vi "Get_Data_Base_file_code.vi"(0 "Results Filename":path, 1 "Data Type":string="Measurement") -> (2 "DB file code":string, 3 "Raw Data Folder":string, 4 "Raw Data File Name":path, 5 "Raw Data File Number":string)   [LabVIEW 2010]
uses:
  Get_File_Code_case.ctl
  Controls/Post_Process.ctl
  Globals/Constants_global.vi
  Globals/Trav_pos_global.vi
  Globals/Meas_global.vi
panel:
  out "File Code Case":T1
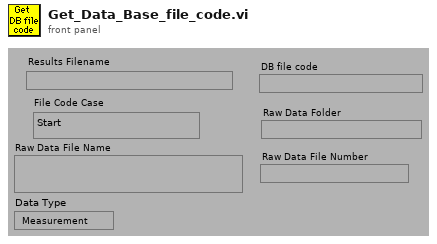
[diagram p1: front panel]
types:
  T1 = typedef "Get_File_Code_case.ctl" = enum16{"Start", "Read DB info file", "Does Results file already exist", "Create DB info directory", "Add file to list", "Write DB info file", "End"}
  T2 = typedef "Post_Process.ctl" = enum16{"Take New Data", "Post Process Raw Data File"}
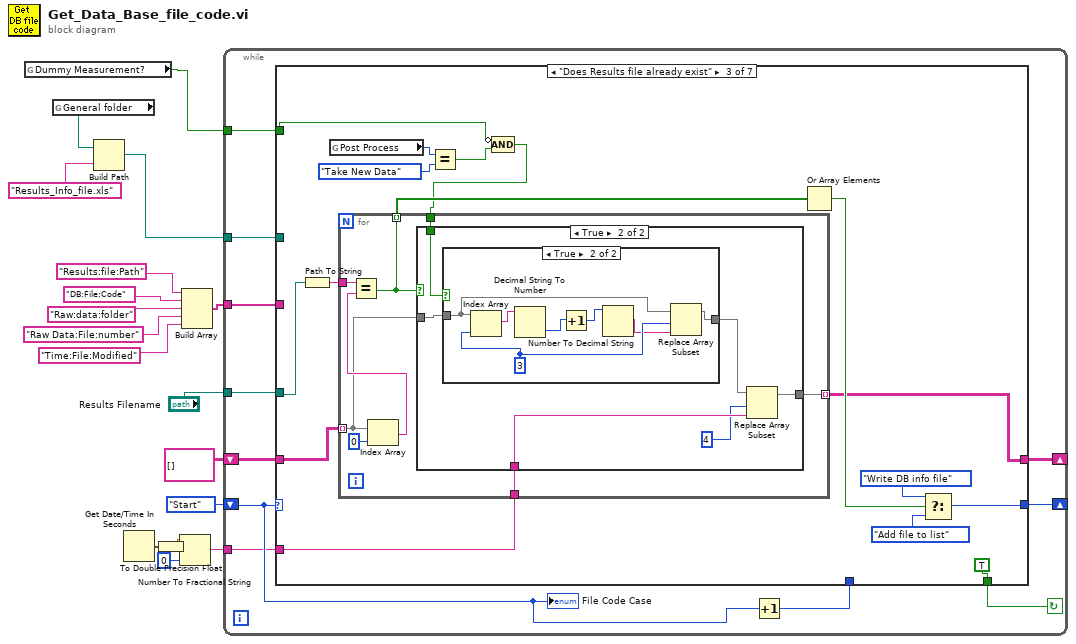
[diagram p0: block diagram]
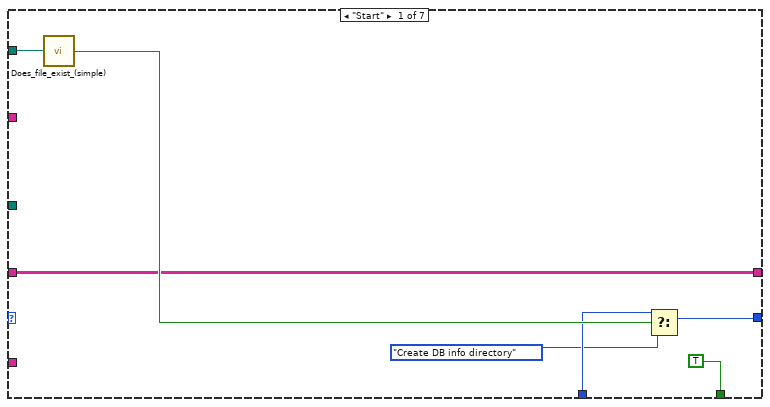
[diagram p2: hidden frame]
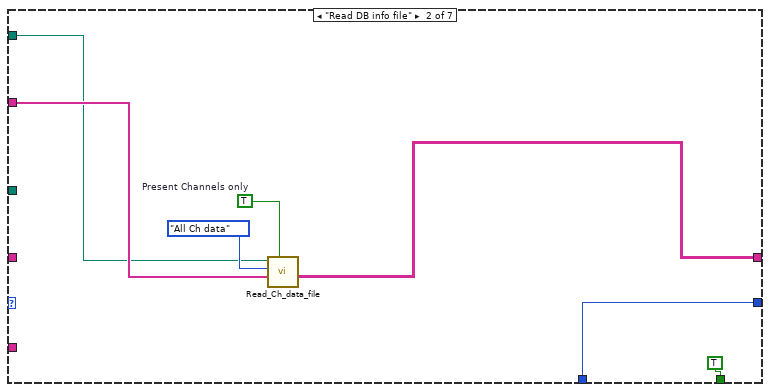
[diagram p3: hidden frame]
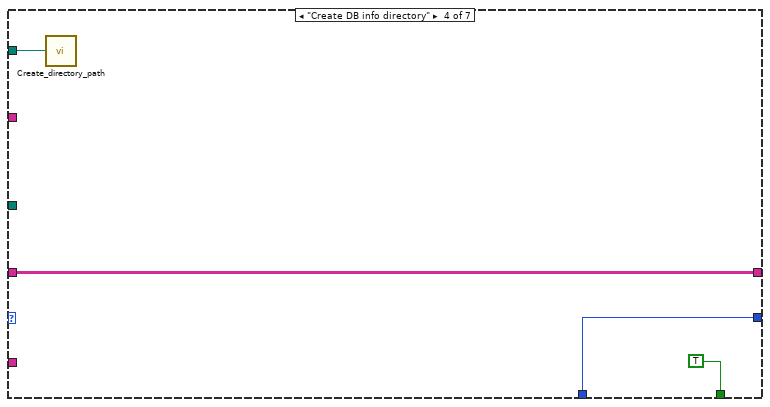
[diagram p6: hidden frame]
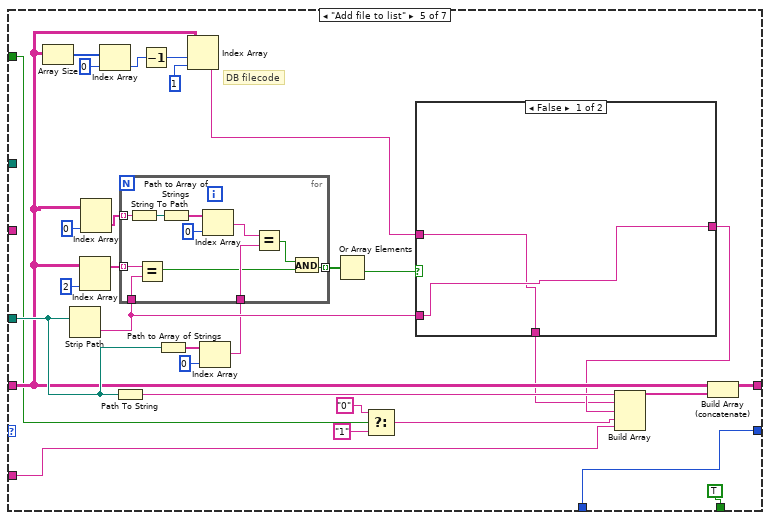
[diagram p7: hidden frame]
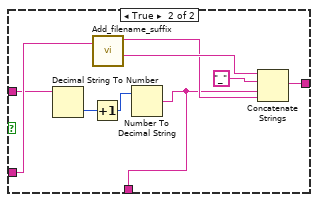
[diagram p8: hidden frame]
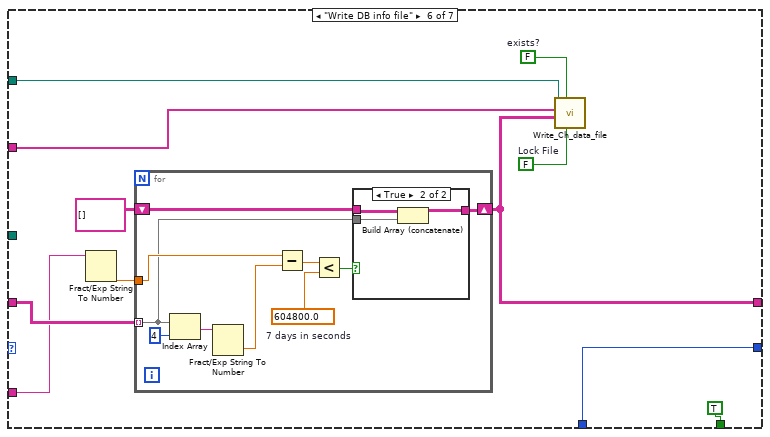
[diagram p9: hidden frame]
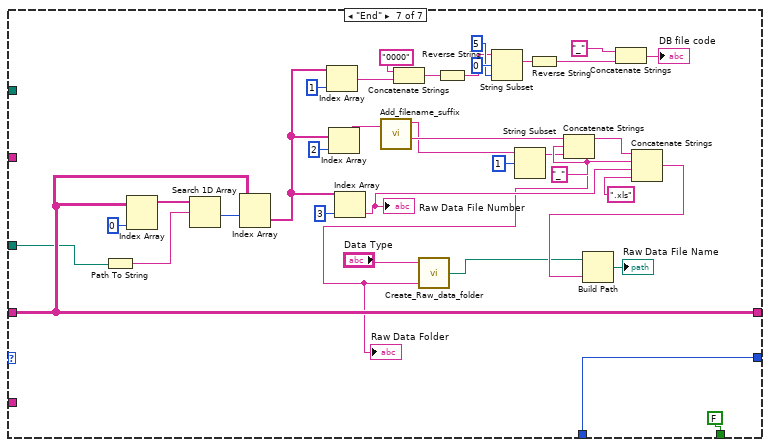
[diagram p11: hidden frame]
diagram:
  n1 = global read "Trav_pos_global.vi" "Dummy Measurement?"() -> (w1:bool)
  n2 = global read "Constants_global.vi" "General folder"() -> (w7:path)
  n3 = Build Path(base path=w7, name or relative path="Results_Info_file.xls" ("Substring")) -> (appended path=w6:path)
  n4 = Get Date/Time In Seconds() -> (seconds since 1Jan1904=w2:timestamp)
  n5 = To Double Precision Float(number=w2) -> (double precision float=w4:dbl)
  n6 = Number To Fractional String(number=w4, precision (6)=i16 0) -> (F-format string=w3:string)  [unwired: 2 out]
  n7 = Build Array("Results:file:Path", "DB:File:Code", "Raw:data:folder", "Raw Data:File:number", "Time:File:Modified") -> (w11:string[])
  n8 = while {
    tunnel: w3 -> [w19]
    tunnel: w11 -> [w20]
    tunnel: "Results Filename" -> [w22]
    shift-left: string[][] [] ("2D data array") -> [w21]
    shift-right: [w23] -> _
    tunnel: w6 -> [w24]
    shift-left: Get_File_Code_case."Start" ("File Code Case") -> [w27]
    shift-right: [w25] -> _
    tunnel: w1 -> [w18]
    stop <- w28 continue-if-true
    n9 = Increment(x=w27) -> (x+1=w26:T1)
    n10 = case shown="\"Does Results file already exist\"" w27 {
      tunnel: [TRUE TRUE TRUE TRUE TRUE TRUE FALSE] -> w28
      tunnel: w26 -> [w32 w42 _ w84 w107 w148 w197]
      tunnel: [w30 w42 w52 w84 w107 w148 w197] -> w25
      tunnel: w24 -> [w34 w36 _ w83 _ w145 _]
      tunnel: [w29 w37 w51 w82 w108 w139 w192] -> w23
      tunnel: w22 -> [_ _ w57 _ w101 _ w179]
      tunnel: w21 -> [w29 _ w58 w82 w96 w143 w192]
      tunnel: w20 -> [_ w40 _ _ _ w146 _]
      tunnel: w19 -> [_ _ w49 _ w105 w142 _]
      tunnel: w18 -> [_ _ w43 _ w92 _ _]
      frame "Start" {
        n11 = call "Does_file_exist_(simple).vi"("Pathname"=w34) -> ("exists?"=w33:bool)
        n12 = Select(t=w32, s=w33, f=Get_File_Code_case."Create DB info directory" ("File Code Case")) -> (s? t:f=w30:T1)
      }
      frame "Read DB info file" {
        w38 = TRUE  # Present Channels only
        n13 = call "Read_Ch_data_file.vi"("Present Channels only"=w38, "Present Channels"=w40, "Output"=enum16{"All Ch data", "The last few rows"}."All Ch data", "Filename"=w36) -> ("Channel Values"=w37:string[][])  [unwired: 1 in, 4 out]
      }
      frame "Does Results file already exist" {
        n14 = Path To String(path=w57) -> (string=w48:string)
        n15 = global read "Meas_global.vi" "Post Process"() -> (w46:T2)
        n16 = Equal?(x=w46, y=Post_Process."Take New Data" ("Post Process")) -> (x = y?=w45:bool)
        n17 = Compound Arithmetic op=AND(invert w43, w45) -> (w44:bool)
        n18 = for {
          tunnel: w58 -> [w63] mode=indexing
          tunnel: w48 -> [w65]
          tunnel: [w62] -> w56 mode=indexing
          tunnel: [w61] -> w51 mode=indexing
          tunnel: w49 -> [w60]
          tunnel: w44 -> [w59]
          n19 = Index Array(array=w63, index=0 ("Index")) -> (element=w64:string)
          n20 = Equal?(x=w65, y=w64) -> (x = y?=w62:bool)
          n21 = case shown="True" w62 {
            tunnel: w63 -> [w67 w73]
            tunnel: [w67 w69] -> w61
            tunnel: w60 -> [_ w71]
            tunnel: w59 -> [_ w68]
            frame False {
            }
            frame True {
              n22 = case shown="True" w68 {
                tunnel: w73 -> [w74 w75]
                tunnel: [w74 w77] -> w72
                frame False {
                }
                frame True {
                  w81 = 3 ("Index")
                  n23 = Index Array(array=w75, index=w81) -> (element=w80:string)
                  n24 = Decimal String To Number(string=w80) -> (number=w79:i32)  [unwired: 3 out]
                  n25 = Increment(x=w79) -> (x+1=w78:i32)
                  n26 = Number To Decimal String(number=w78) -> (decimal integer string=w76:string)  [unwired: 1 out]
                  n27 = Replace Array Subset(array=w75, new element=w76, index=w81) -> (w77:string[])
                }
              }
              n28 = Replace Array Subset(array=w72, new element=w71, index=4 ("Index")) -> (w69:string[])
            }
          }
        }
        n29 = Or Array Elements(Boolean array=w56) -> (logical OR=w55:bool)
        n30 = Select(t=Get_File_Code_case."Write DB info file" ("File Code Case"), s=w55, f=Get_File_Code_case."Add file to list" ("File Code Case")) -> (s? t:f=w52:T1)
      }
      frame "Create DB info directory" {
        n31 = call "Create_directory_path.vi"("Path name"=w83) -> ()  [unwired: 1 out]
      }
      frame "Add file to list" {
        # "DB filecode"
        n32 = Array Size(array=w96) -> (size(s)=w113:i32[])
        n33 = Strip Path(path=w101) -> (name=w99:string)  [unwired: 1 out]
        n34 = Index Array(array=w96, index (col)=2) -> (element=w98:string[])  [unwired: 1 in]
        n35 = Index Array(array=w96, index (col)=0) -> (element=w97:string[])  [unwired: 1 in]
        n36 = Index Array(array=w113, index=0) -> (element=w112:i32)
        n37 = Path To String(path=w101) -> (string=w104:string)
        n38 = Decrement(x=w112) -> (x-1=w111:i32)
        n39 = Path to Array of Strings(0:w101) -> (2:w102:string[])  [unwired: 1 out]
        n40 = Index Array(array=w96, index (row)=w111, index (col)=1) -> (element=w87:string)
        n41 = Index Array(array=w102, index=0 ("Index")) -> (element=w95:string)
        n42 = for {
          tunnel: w99 -> [w126]
          tunnel: w98 -> [w125] mode=indexing
          tunnel: w97 -> [w121] mode=indexing
          tunnel: w95 -> [w119]
          tunnel: [w116] -> w94 mode=indexing
          n43 = String To Path(string=w121) -> (path=w122:path)
          n44 = Equal?(x=w125, y=w126) -> (x = y?=w117:bool)
          n45 = Path to Array of Strings(0:w122) -> (2:w123:string[])  [unwired: 1 out]
          n46 = Index Array(array=w123, index=0 ("Index")) -> (element=w120:string)
          n47 = Equal?(x=w120, y=w119) -> (x = y?=w118:bool)
          n48 = And(x=w118, y=w117) -> (x .and. y?=w116:bool)
        }
        n49 = Or Array Elements(Boolean array=w94) -> (logical OR=w93:bool)
        n50 = Select(t="0", s=w92, f="1") -> (s? t:f=w89:string)
        n51 = case shown="False" w93 {
          tunnel: w87 -> [w127 w130]
          tunnel: [w128 w137] -> w88
          tunnel: w99 -> [w128 w135]
          tunnel: [w127 w129] -> w86
          frame False {
          }
          frame True {
            n52 = Decimal String To Number(string=w130) -> (number=w131:i32)  [unwired: 3 out]
            n53 = Increment(x=w131) -> (x+1=w132:i32)
            n54 = call "Add_filename_suffix.vi"("Filename"=w135) -> ("Original Suffix"=w133:string, "Base name"=w134:string)  [unwired: 1 in, 2 out]
            n55 = Number To Decimal String(number=w132) -> (decimal integer string=w129:string)  [unwired: 1 out]
            n56 = Concatenate Strings(w134, "_" ("Substring"), w129, w133) -> (w137:string)
          }
        }
        n57 = Build Array(w104, w86, w88, w89, w105) -> (w109:string[])
        n58 = Build Array (concatenate)(w96, w109) -> (w108:string[][])
      }
      frame "Write DB info file" {
        w138 = FALSE  # Lock File
        w144 = FALSE  # exists?
        n59 = Fract/Exp String To Number(string=w142) -> (number=w141:dbl)  [unwired: 4 out]
        n60 = for {
          shift-right: [w151] -> w139
          shift-left: string[][] [] -> [w150]
          tunnel: w143 -> [w149] mode=indexing
          tunnel: w141 -> [w156]
          w153 = 604800.0  # 7 days in seconds
          n61 = Index Array(array=w149, index=4 ("Index")) -> (element=w157:string)
          n62 = Fract/Exp String To Number(string=w157) -> (number=w155:dbl)  [unwired: 4 out]
          n63 = Subtract(x=w156, y=w155) -> (x-y=w154:dbl)
          n64 = Less?(x=w154, y=w153) -> (x < y?=w152:bool)
          n65 = case shown="True" w152 {
            tunnel: [w159 w161] -> w151
            tunnel: w150 -> [w159 w162]
            tunnel: w149 -> [_ w160]
            frame False {
            }
            frame True {
              n66 = Build Array (concatenate)(w162, w160) -> (w161:string[][])
            }
          }
        }
        n67 = call "Write_Ch_data_file.vi"("Lock File"=w138, "exists?"=w144, "Channel Values"=w139, "Channel names"=w146, "Filename"=w145) -> ()  [unwired: 3 in, 4 out]
      }
      frame "End" {
        w167 = "_" ("Substring")
        n68 = Path To String(path=w179) -> (string=w178:string)
        n69 = Index Array(array=w192, index (col)=0) -> (element=w194:string[])  [unwired: 1 in]
        n70 = Search 1D Array(1D array=w194, element=w178) -> (index of element=w193:i32)  [unwired: 1 out]
        n71 = Index Array(array=w192, index (row)=w193) -> (element=w177:string[])  [unwired: 1 in]
        n72 = Index Array(array=w177, index=1 ("Index")) -> (element=w184:string)
        n73 = Index Array(array=w177, index=2 ("Index")) -> (element=w169:string)
        n74 = Index Array(array=w177, index=3 ("Index")) -> (element=w173:string)
        "Raw Data File Number" <- w173
        n75 = call "Add_filename_suffix.vi"("Filename"=w169) -> ("Original Suffix"=w164:string, "Base name"=w168:string)  [unwired: 1 in, 2 out]
        n76 = Concatenate Strings("0000", w184) -> (w180:string)
        n77 = Reverse String(1:w180) -> (0:w181:string)
        n78 = String Subset(string=w181, offset (0)=0, length (rest)=5 ("length")) -> (substring=w182:string)
        n79 = String Subset(string=w164, offset (0)=1) -> (substring=w166:string)  [unwired: 1 out]
        n80 = Reverse String(1:w182) -> (0:w183:string)
        n81 = Concatenate Strings(w168, w167, w166) -> (w165:string)
        "Raw Data Folder" <- w165
        n82 = call "Create_Raw_data_folder.vi"("Folder Name"=w165, "Data Type"="Data Type") -> ("Raw Data Folder"=w171:path)  [unwired: 1 in]
        n83 = Concatenate Strings("_" ("Substring"), w183) -> (→"DB file code":string)
        n84 = Concatenate Strings(w168, w167, w173, ".xls" ("string")) -> (w174:string)
        n85 = Build Path(base path=w171, name or relative path=w174) -> (appended path=→"Raw Data File Name":path)
      }
    }
    "File Code Case" <- w27
  }
